vi "Destroy.vi"(11 "Ex Event Actor in":refnum<class "Ex Event Actor.lvclass">) -> (3 "Ex Event Actor out":refnum<class "Ex Event Actor.lvclass">)   [LabVIEW 2021, in "Ex Event Actor.lvlib" / "Ex Event Actor.lvclass"]
uses:
  Ex Event Actor.lvclass
  Ex Event Actor.lvclass/Ex Event Actor.ctl
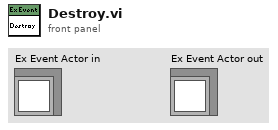
[diagram p1: front panel]
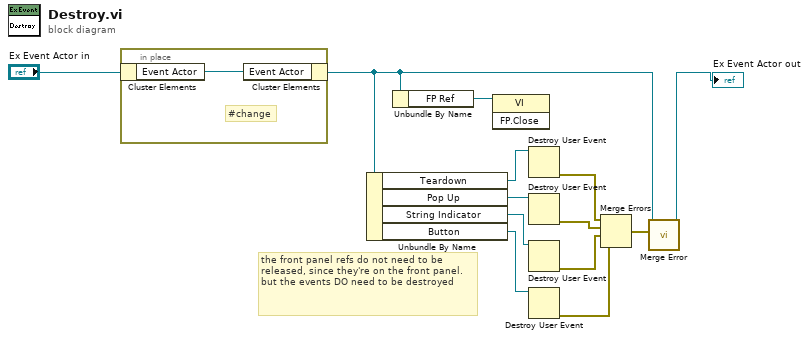
[diagram p0: block diagram]
diagram:
  # "the front panel refs do not need to be released, since they're on the front panel. but the events DO need to be destroyed"
  n1 = in-place {
    # "#change"
    n2 = in-place-cluster #1("Ex Event Actor in") -> ("Event Actor"=w14:refnum<class "Event Actor.lvclass">)
    n3 = in-place-cluster #1("Event Actor"=w14) -> (w2:refnum<class "Ex Event Actor.lvclass">)
  }
  n4 = Unbundle By Name(w2) -> ("Teardown"=w13:refnum<user-event>, "Pop Up"=w12:refnum<user-event>, "String Indicator"=w11:refnum<user-event>, "Button"=w10:refnum<user-event>)
  n5 = Unbundle By Name(w2) -> ("FP Ref"=w9:refnum<vi>)
  n6 = invoke class="VI" method="FP.Close"(reference=w9) -> ()  [unwired: 2 in, 3 out]
  n7 = Destroy User Event(user event=w13) -> (error out=w8:errorcluster)  [unwired: 1 in]
  n8 = Destroy User Event(user event=w12) -> (error out=w7:errorcluster)  [unwired: 1 in]
  n9 = Destroy User Event(user event=w11) -> (error out=w6:errorcluster)  [unwired: 1 in]
  n10 = Destroy User Event(user event=w10) -> (error out=w5:errorcluster)  [unwired: 1 in]
  n11 = Merge Errors(w8, w7, w6, w5) -> (w4:errorcluster)
  n12 = call-dynamic "Merge Error.vi"("Error"=w4, "Ex Event Actor in"=w2) -> ("Ex Event Actor out"=→"Ex Event Actor out":refnum<class "Ex Event Actor.lvclass">)  [unwired: 9 in]
